vi "Append Control Value.vi"(9 "Value":variant, 10 "Name":string, 11 "Control Values":cluster{"Name":string, "Value":variant}[](array[cluster])) -> (3 "Control Values":cluster{"Name":string, "Value":variant}[](array[cluster]))   [LabVIEW 2020, in "Mock Class Generator.lvclass"]
uses:
  Mock Class Generator.lvclass
  Mock Class Generator.lvclass/Mock Class Generator.ctl
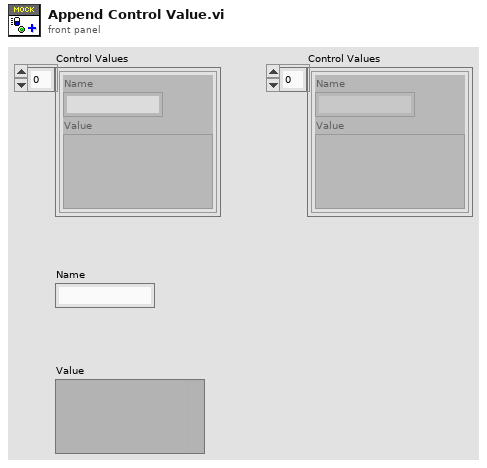
[diagram p1: front panel]
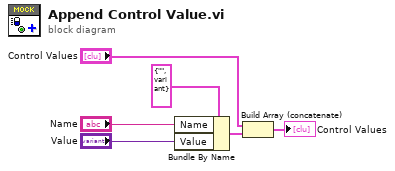
[diagram p0: block diagram]
diagram:
  n1 = Bundle By Name(cluster=cluster{"Name":string, "Value":variant} {"Name"="", "Value"=variant} ("element"), "Name"="Name", "Value"="Value") -> (w4:cluster{"Name":string, "Value":variant})
  n2 = Build Array (concatenate)("Control Values", w4) -> (→"Control Values":cluster{"Name":string, "Value":variant}[])
